vi "Read ADXL345.vi"(10 "Private Data In":T1) -> (0 "Z (g)":fxp<+/-,32,10>, 1 "Y (g)":fxp<+/-,32,10>, 2 "X (g)":fxp<+/-,32,10>, 3 "Private Data Out":T1)   [LabVIEW 2014]
uses:
  <vilib>/IEDriver/SPIandI2C/FPGA/Type Def/Private Data (SPI).ctl
  SPI Parameters.ctl
  <vilib>/IEDriver/SPIandI2C/FPGA/Library/IP SPI&I2C.lvlib
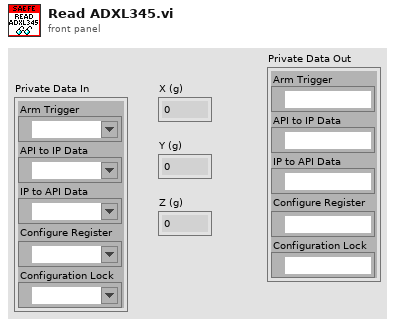
[diagram p1: front panel]
types:
  T1 = typedef "IP SPI&I2C.lvlib/Private Data (SPI).ctl" = cluster{"Arm Trigger":refnum<k21>, "API to IP Data":refnum<k21>, "IP to API Data":refnum<k21>, "Configure Register":refnum<k21>, "Configuration Lock":refnum<k21>}
  T2 = typedef "SPI Parameters.ctl" = cluster{"Clock Divider":u32, "Mode":u8, "CS Active State":bool}
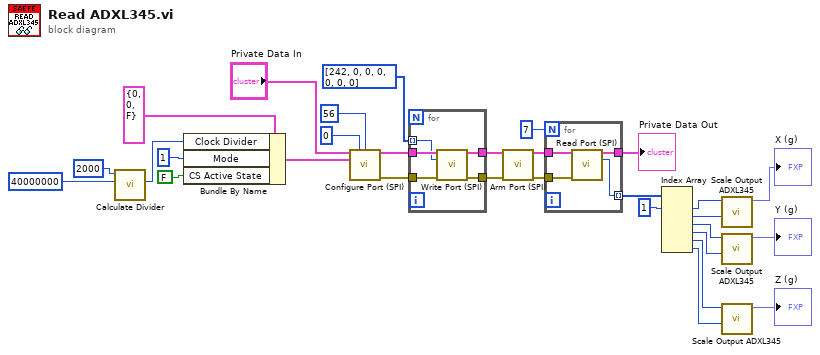
[diagram p0: block diagram]
diagram:
  n1 = call <vilib>:"Calculate Divider.vi"("FPGA Clock (Hz)"=u32 40000000 ("Clock Rate (Hz)"), "Clock Rate (Hz)"=u32 2000) -> ("Clock Divider"=w4:u32)  [unwired: 7 in, 2 out]
  n2 = Bundle By Name(cluster=T2 {"Clock Divider"=0, "Mode"=0, "CS Active State"=FALSE} ("SPI Parameters"), "Clock Divider"=w4, "Mode"=u8 1, "CS Active State"=FALSE) -> (w6:T2)
  n3 = call <vilib>:"Configure Port (SPI).vi"("Private Data In"="Private Data In", "Chip Select"=u8 0, "Number of Bits"=u16 56, "SPI Parameters"=w6) -> ("Private Data Out"=w10:T1, "error out"=w11:errorcluster)  [unwired: 9 in, 1 out]
  n4 = for {
    tunnel: u8[] [242, 0, 0, 0, 0, 0, 0] ("Write Data") -> [w31] mode=indexing
    tunnel: w10 -> [w35]
    tunnel: [w33] -> w15
    tunnel: w11 -> [w34]
    tunnel: [w32] -> w16
    n5 = call <vilib>:"Write Port (SPI).vi"("Private Data In"=w35, "Data In"=w31, "error in"=w34) -> ("Private Data Out"=w33:T1, "error out"=w32:errorcluster)  [unwired: 10 in, 1 out]
  }
  n6 = call <vilib>:"Arm Port (SPI).vi"("Private Data In"=w15, "error in"=w16) -> ("Private Data Out"=w18:T1, "error out"=w19:errorcluster)  [unwired: 11 in, 1 out]
  n7 = for {
    N: 7 -> [_]
    tunnel: w18 -> [w39]
    tunnel: w19 -> [w38]
    tunnel: [w37] -> w20 mode=indexing
    tunnel: [w36] -> w1
    n8 = call <vilib>:"Read Port (SPI).vi"("Private Data In"=w39, "error in"=w38) -> ("Private Data Out"=w36:T1, "Data Out"=w37:u8)  [unwired: 10 in, 2 out]
  }
  "Private Data Out" <- w1
  n9 = Index Array(array=w20, index #1=1 ("index")) -> (element #1=w22:u8, element #2=w23:u8, element #3=w24:u8, element #4=w25:u8, element #5=w26:u8, element #6=w27:u8)  [unwired: 5 in]
  n10 = call "Scale Output ADXL345.vi"("Byte1"=w23, "Byte0"=w22) -> ("G's"=→"X (g)":fxp<+/-,32,10>)  [unwired: 9 in]
  n11 = call "Scale Output ADXL345.vi"("Byte1"=w25, "Byte0"=w24) -> ("G's"=→"Y (g)":fxp<+/-,32,10>)  [unwired: 9 in]
  n12 = call "Scale Output ADXL345.vi"("Byte1"=w27, "Byte0"=w26) -> ("G's"=→"Z (g)":fxp<+/-,32,10>)  [unwired: 9 in]
